vi "Search Keywords.vi"(9 "Delimiter":string=" ", 10 "Keyword Array":string[](array[string]), 11 "Str Refnum":refnum<vi>) -> (0 "Match Found?":bool, 1 "Match Cluster":cluster{"Item Index":i32, "Offset":i32}, 2 "Keyword Array Out":string[](array[string]), 3 "Str Refnum Out":refnum<vi>)   [LabVIEW 2011, in "Intellisense Xcontrol.xctl"]
uses:
  Intellisense Xcontrol.xctl
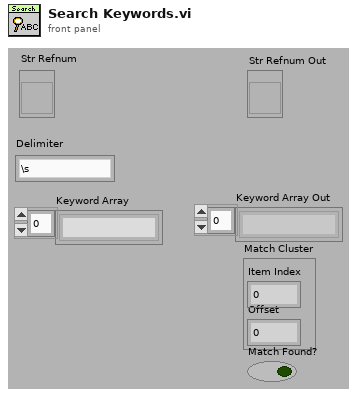
[diagram p1: front panel]
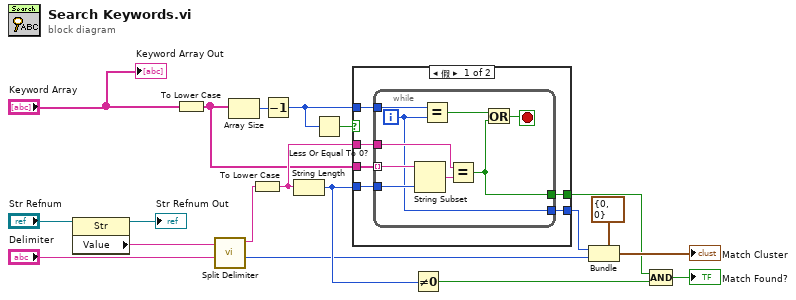
[diagram p0: block diagram]
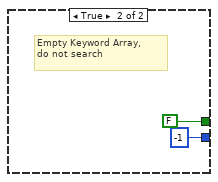
[diagram p2: hidden frame]
diagram:
  n1 = property class="Str"(reference="Str Refnum") -> (reference out=→"Str Refnum Out":refnum<vi>, "Value"=w2:string)  [unwired: 1 in, 1 out]
  n2 = To Lower Case(string="Keyword Array") -> (all lower case string=w5:string[])
  n3 = call "Split Delimiter.vi"("Delimiter"="Delimiter", "String In"=w2) -> ("Offset"=w3:i32, "After Delimiter"=w4:string)  [unwired: 8 in]
  n4 = Array Size(array=w5) -> (size(s)=w9:i32)
  n5 = To Lower Case(string=w4) -> (all lower case string=w8:string)
  n6 = Decrement(x=w9) -> (x-1=w6:i32)
  n7 = String Length(string=w8) -> (length=w13:i32)
  n8 = Less Or Equal To 0?(x=w6) -> (x <= 0?=w7:bool)
  n9 = case shown="假" w7 {
    tunnel: w13 -> [w25 _]
    tunnel: [w24 -1] -> w12
    tunnel: [w23 FALSE] -> w10
    tunnel: w6 -> [w22 _]
    tunnel: w8 -> [w21 _]
    tunnel: w5 -> [w20 _]
    frame False {
      n10 = while {
        tunnel: w21 -> [w33]
        tunnel: w20 -> [w30] mode=indexing
        tunnel: w25 -> [w28]
        tunnel: w22 -> [w29]
        tunnel: [w26] -> w23
        tunnel: [w27] -> w24
        i -> [w27]
        stop <- w32 stop-if-true
        n11 = String Subset(string=w30, length (rest)=w28) -> (substring=w34:string)  [unwired: 1 in]
        n12 = Equal?(x=w29, y=w27) -> (x = y?=w31:bool)
        n13 = Equal?(x=w33, y=w34) -> (x = y?=w26:bool)
        n14 = Or(x=w31, y=w26) -> (x .or. y?=w32:bool)
      }
    }
    frame True {
      # "Empty Keyword Array,\ndo not search"
    }
  }
  n15 = Not Equal To 0?(x=w13) -> (x != 0?=w14:bool)
  n16 = Bundle(cluster=cluster{"Item Index":i32, "Offset":i32} {"Item Index"=0, "Offset"=0}, "Item Index"=w12, "Offset"=w3) -> (→"Match Cluster":cluster{"Item Index":i32, "Offset":i32})
  n17 = Compound Arithmetic op=AND(w10, w14) -> (→"Match Found?":bool)
  "Keyword Array Out" <- "Keyword Array"
